vi "LeerArchivoConfiguracion.vi"(8 "error in":errorcluster, 11 "Prueba31 in":refnum<class "Prueba21.lvclass">) -> (0 "error out":errorcluster, 3 "Prueba31 out":refnum<class "Prueba21.lvclass">)   [LabVIEW 2019, in "Prueba21.lvclass"]
uses:
  Prueba21.lvclass
  Prueba21.lvclass/Prueba21.ctl
  <vilib>/Utility/config.llb/Read Key (Boolean).vi
  <vilib>/Utility/config.llb/Read Key (String).vi
  <vilib>/Utility/config.llb/NI_LVConfig.lvlib
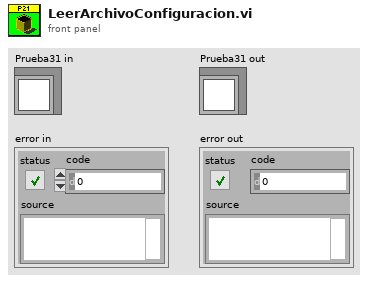
[diagram p1: front panel]
types:
  T1 = typedef "NI_LVConfig.lvlib/Config Data RefNum.ctl" = refnum<k1>
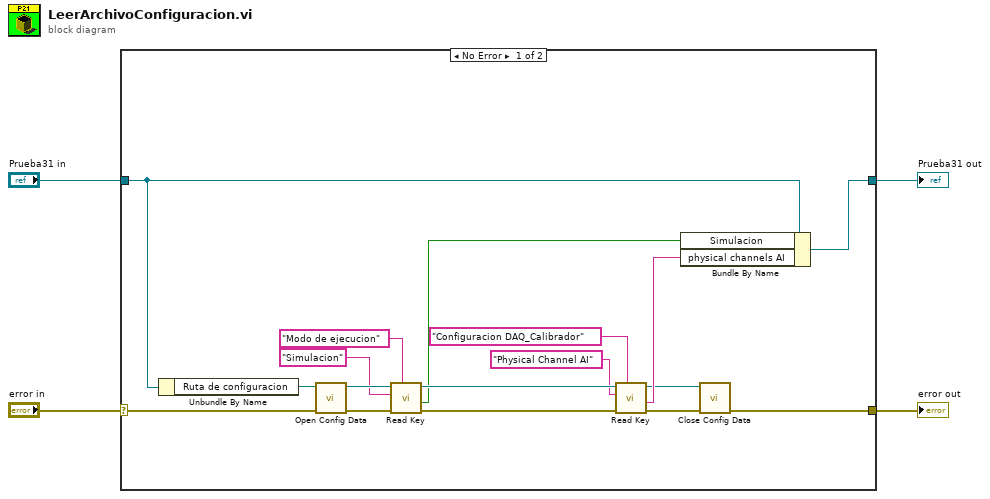
[diagram p0: block diagram]
diagram:
  n1 = case shown="No Error" "error in" {
    selector: "error in" -> [w21 w22]
    tunnel: [w10 w22] -> w2
    tunnel: [w8 w23] -> w4
    tunnel: "Prueba31 in" -> [w7 w23]
    frame No Error {
      n2 = Unbundle By Name(w7) -> ("Ruta de configuracion"=w20:path)
      n3 = call <vilib>:"Open Config Data.vi"("error in (no error)"=w21, "configuration file path"=w20) -> ("error out"=w19:errorcluster, "refnum"=w18:T1)  [unwired: 7 in, 1 out]
      n4 = call-poly <vilib>:"Read Key.vi"("section"="Modo de ejecucion", "error in (no error)"=w19, "key"="Simulacion", "refnum"=w18) -> ("error out"=w14:errorcluster, "value"=w13:bool, "refnum out"=w16:T1)  [unwired: 4 in, 1 out]
      n5 = call-poly <vilib>:"Read Key.vi"("section"="Configuracion DAQ_Calibrador", "error in (no error)"=w14, "key"="Physical Channel AI", "refnum"=w16) -> ("error out"=w11:errorcluster, "value"=w12:string, "refnum out"=w9:T1)  [unwired: 4 in, 1 out]
      n6 = Bundle By Name(cluster=w7, "Simulacion"=w13, "physical channels AI"=w12) -> (w8:refnum<class "Prueba21.lvclass">)
      n7 = call <vilib>:"Close Config Data.vi"("error in (no error)"=w11, "refnum"=w9) -> ("error out"=w10:errorcluster)  [unwired: 8 in, 1 out]
    }
    frame Error {
    }
  }
  "Prueba31 out" <- w4
  "error out" <- w2
